vi "Set Initial Orientation.vi"(8 "Error In":errorcluster, 10 "Initial Orientation":T1=1 items=["Horizontal"=1, "Vertical"=2], 11 "Splitter Builder in":refnum<class "Splitter Builder.lvclass">) -> (0 "Error Out":errorcluster, 3 "Splitter Builder out":refnum<class "Splitter Builder.lvclass">)   [LabVIEW 2014, in "Splitter Builder.lvclass"]
doc: "Specifies the splitter orientation to use when calling Create Container.vi.\n\n\nCopyright (c) 2019 Sze Howe Koh.\nThis code is licensed under the MIT license."
uses:
  Splitter Builder.lvclass
  <vilib>/addons/LQ/LQ Core/Qt/Orientation.ctl
  Splitter Builder.lvclass/Splitter Builder.ctl
  <vilib>/addons/LQ/LQ Core/Qt/Qt.lvlib
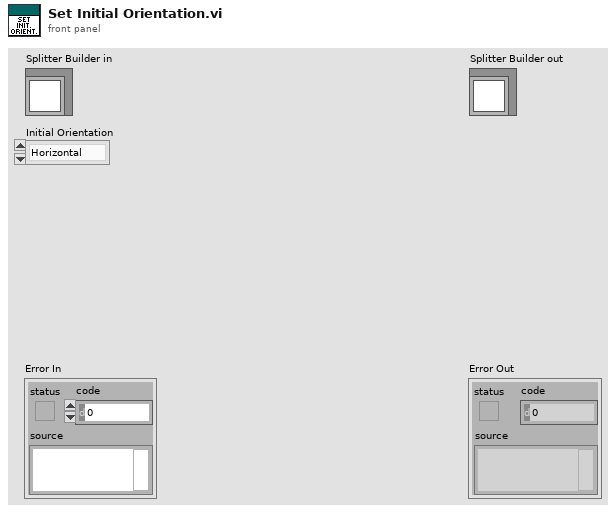
[diagram p1: front panel]
types:
  T1 = typedef "Qt.lvlib/Orientation.ctl" = i32
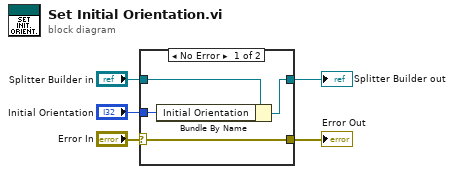
[diagram p0: block diagram]
diagram:
  n1 = case shown="No Error" "Error In" {
    selector: "Error In" -> [w9 w10]
    tunnel: [w9 w10] -> w4
    tunnel: [w7 w11] -> w2
    tunnel: "Splitter Builder in" -> [w8 w11]
    tunnel: "Initial Orientation" -> [w6 _]
    frame No Error {
      n2 = Bundle By Name(cluster=w8, "Initial Orientation"=w6) -> (w7:refnum<class "Splitter Builder.lvclass">)
    }
    frame Error {
    }
  }
  "Error Out" <- w4
  "Splitter Builder out" <- w2
